vi "Handle Command.vi"(8 "error in (no error)":errorcluster, 9 "Data":variant, 10 "Command":string, 11 "Inst.Attocube-3DR in":refnum<class "Inst.Attocube-3DR.lvclass">) -> (0 "error out":errorcluster, 1 "Processed Data":variant, 2 "Command":string, 3 "Inst.Attocube-3DR out":refnum<class "Inst.Attocube-3DR.lvclass">)   [LabVIEW 2019, in "Inst.Attocube-3DR.lvclass"]
uses:
  Inst.Attocube-3DR.lvclass
  Inst.Attocube-3DR.lvclass/Inst.Attocube-3DR.ctl
  Typedefs/Inst.Attocube-3DR.getAll--Cluster.ctl
  9aec49fd-fe04-463a-be35-b7075f22e824.vi
  9aec49fd-fe04-463a-be35-b7075f22e824.vi/2713e523-c1ef-4f5d-940a-2c453df62ff4.vi
  9aec49fd-fe04-463a-be35-b7075f22e824.vi/a90875ce-4e03-4b08-b88d-0b37294445d5.vi
  <vilib>/Utility/Data Type/Get Type Information.vi
  <vilib>/JDP Science/JSONtext/JSON text to Variant.vi
  <vilib>/JDP Science/JSONtext/LVClass Serializer/JSONtext LVClass Serializer.lvclass
  <userlib>/LevyLab/Instrument Framework/Instrument Types/VSource/Instrument.VSource.lvclass
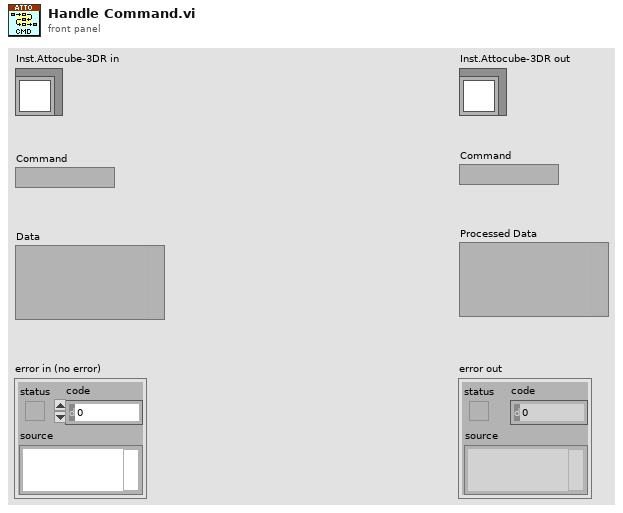
[diagram p1: front panel]
types:
  T1 = typedef "Inst.Attocube-3DR.lvclass/Inst.Attocube-3DR.getAll--Cluster.ctl" = cluster{"Axis 1: Amplitude":i32, "Axis 1: Capacitance":i32, "Axis 1: Current Position":i32, "Axis 1: DCLevel":i32, "Axis 1: Frequency":i32, "Axis 1: StepWidth":i32, "Axis 1: control mode":i32, "Axis 1: rot. count":i32, "Axis 1: sp position":i32, "Axis 1: sp rot. count":i32, "Axis 1: speed":i32, "Axis 1: Target GND":bool, "Axis 1: Output":bool, "Axis 1: Single Circle Mode":bool, "Axis 1: moving":bool, "Axis 1: stop detected":bool, "Axis 1:  sensor error":bool, "Axis 1: sensor diconnected":bool, "Axis 1: stop enable":bool, "Axis 2: Current Position":i32, "Axis 2: DCLevel":i32, "Axis 2: Frequency":i32, "Axis 2: StepWidth":i32, "Axis 2: control mode":i32, "Axis 2: rot. count":i32, "Axis 2: sp position":i32, "Axis 2: sp rot. count":i32, "Axis 2: speed":i32, "Axis 2: Capacitance":i32, "Axis 2: Amplitude":i32, "Axis 2: Target GND":bool, "Axis 2: Output":bool, "Axis 2: Single Circle Mode":bool, "Axis 2: moving":bool, "Axis 2: stop detected":bool, "Axis 2:  sensor error":bool, "Axis 2: sensor diconnected":bool, "Axis 2: stop enable":bool}
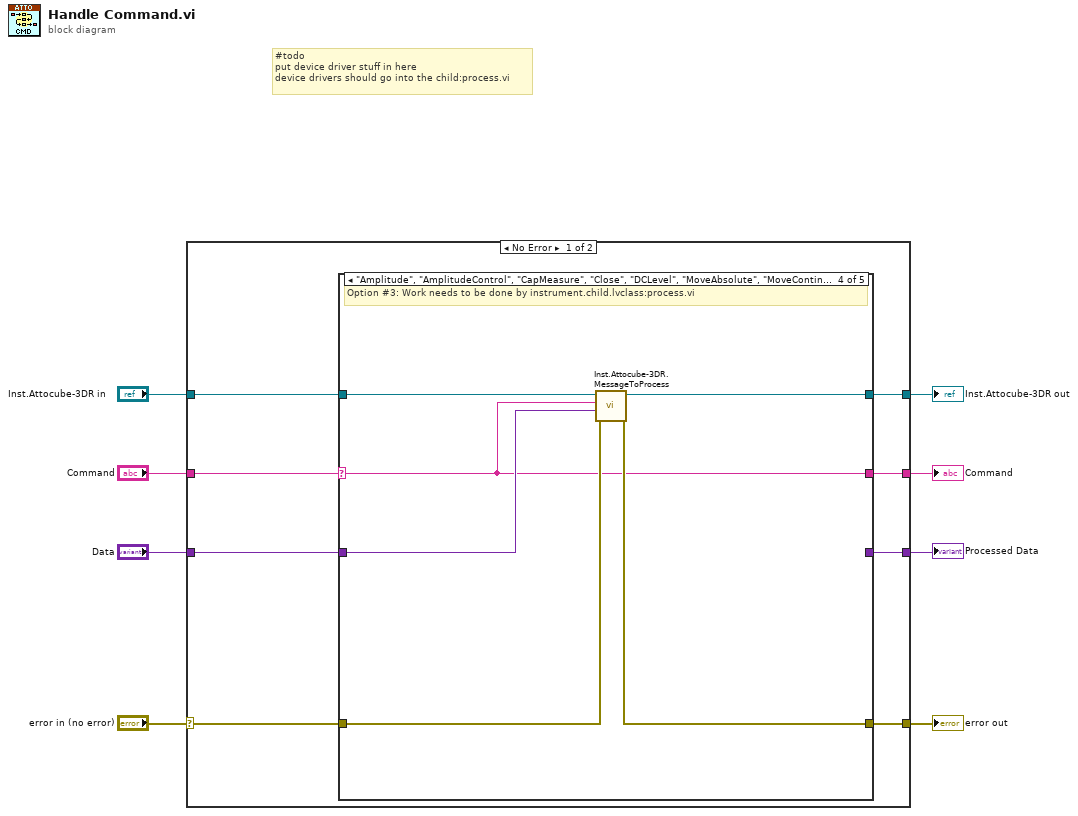
[diagram p0: block diagram]
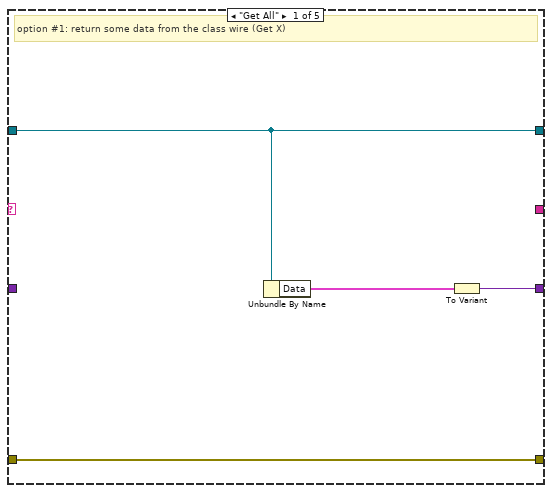
[diagram p2: hidden frame]
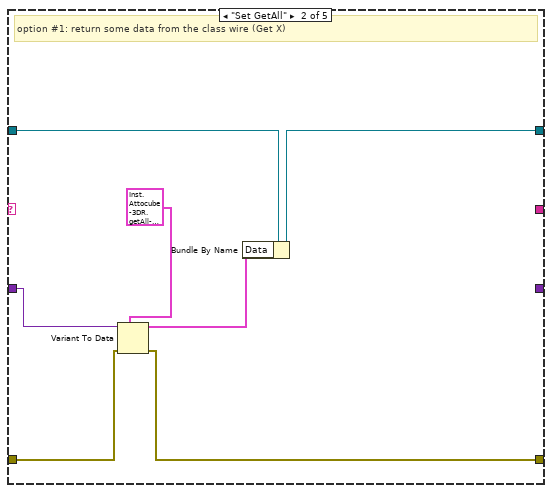
[diagram p3: hidden frame]
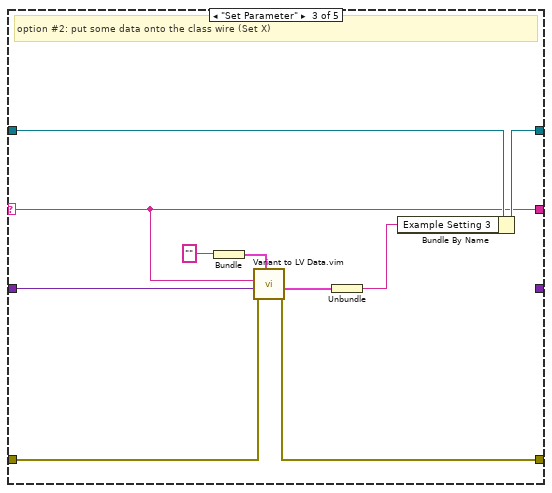
[diagram p4: hidden frame]
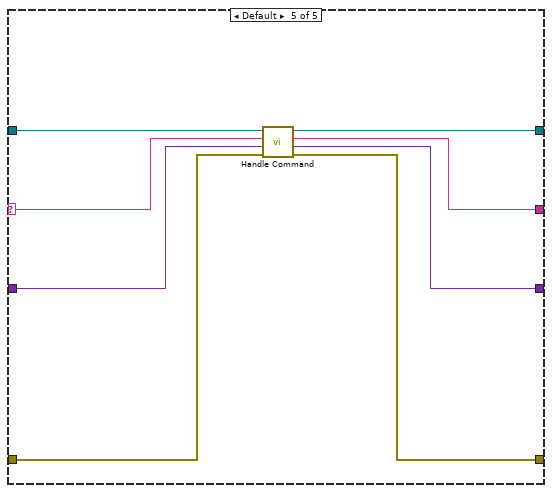
[diagram p5: hidden frame]
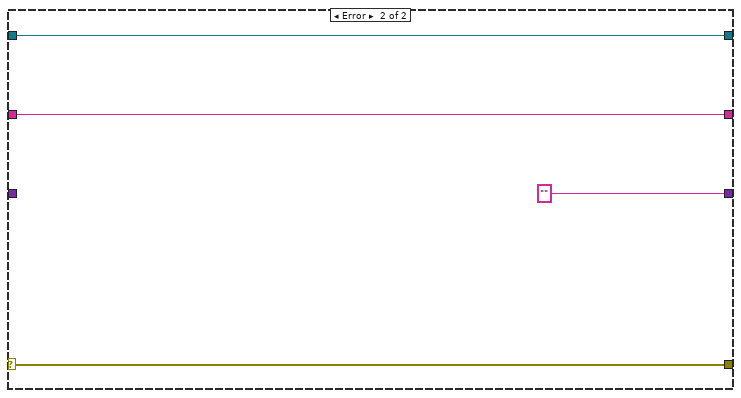
[diagram p6: hidden frame]
diagram:
  # "#todo\nput device driver stuff in here\ndevice drivers should go into the child:process.vi"
  n1 = case shown="No Error" "error in (no error)" {
    selector: "error in (no error)" -> [w10 w55]
    tunnel: [w12 w55] -> w6
    tunnel: [w14 w54] -> w5
    tunnel: "Inst.Attocube-3DR in" -> [w15 w54]
    tunnel: "Command" -> [w16 w52]
    tunnel: [w13 "" ("String")] -> w3
    tunnel: "Data" -> [w9 _]
    tunnel: [w11 w52] -> w1
    frame No Error {
      n2 = case shown="\"Amplitude\", \"AmplitudeControl\", \"CapMeasure\", \"Close\", \"DCLevel\", \"MoveAbsolute\", \"MoveContinuous\", \"MoveRelative\", \"MoveSingleStep\", \"Open\", \"SetOutput\", \"SetTargetGround\", \"SingleCircleMode\", \"StopDetection\", \"StopMoving\", \"setFrequency\"" w16 {
        selector: w16 -> [_ _ w32 w38 w45]
        tunnel: w15 -> [w19 w21 w37 w43 w49]
        tunnel: [w19 w22 w36 w42 w46] -> w14
        tunnel: [w17 _ _ _ w48] -> w13
        tunnel: w10 -> [w18 w26 w35 w41 w50]
        tunnel: w9 -> [_ w25 w33 w39 w51]
        tunnel: [w18 w27 w34 w40 w47] -> w12
        tunnel: [_ _ w32 w38 w44] -> w11
        frame "Get All" {
          # "option #1: return some data from the class wire (Get X)"
          n3 = Unbundle By Name(w19) -> ("Data"=w20:T1)
          n4 = To Variant(anything=w20) -> (Variant=w17:variant)
        }
        frame "Set GetAll" {
          # "option #1: return some data from the class wire (Get X)"
          n5 = Variant To Data(error in=w26, type=T1 {"Axis 1: Amplitude"=0, "Axis 1: Capacitance"=0, "Axis 1: Current Position"=0, "Axis 1: DCLevel"=0, "Axis 1: Frequency"=0, "Axis 1: StepWidth"=0, "Axis 1: control mode"=0, "Axis 1: rot. count"=0, "Axis 1: sp position"=0, "Axis 1: sp rot. count"=0, "Axis 1: speed"=0, "Axis 1: Target GND"=FALSE, "Axis 1: Output"=FALSE, "Axis 1: Single Circle Mode"=FALSE, "Axis 1: moving"=FALSE, "Axis 1: stop detected"=FALSE, "Axis 1:  sensor error"=FALSE, "Axis 1: sensor diconnected"=FALSE, "Axis 1: stop enable"=FALSE, "Axis 2: Current Position"=0, "Axis 2: DCLevel"=0, "Axis 2: Frequency"=0, "Axis 2: StepWidth"=0, "Axis 2: control mode"=0, "Axis 2: rot. count"=0, "Axis 2: sp position"=0, "Axis 2: sp rot. count"=0, "Axis 2: speed"=0, "Axis 2: Capacitance"=0, "Axis 2: Amplitude"=0, "Axis 2: Target GND"=FALSE, "Axis 2: Output"=FALSE, "Axis 2: Single Circle Mode"=FALSE, "Axis 2: moving"=FALSE, "Axis 2: stop detected"=FALSE, "Axis 2:  sensor error"=FALSE, "Axis 2: sensor diconnected"=FALSE, "Axis 2: stop enable"=FALSE} ("getAll"), Variant=w25) -> (data=w23:T1, error out=w27:errorcluster)
          n6 = Bundle By Name(cluster=w21, "Data"=w23) -> (w22:refnum<class "Inst.Attocube-3DR.lvclass">)
        }
        frame "Set Parameter" {
          # "option #2: put some data onto the class wire (Set X)"
          n7 = Bundle("") -> (w30:cluster{string})  [unwired: 1 in]
          n8 = call "Variant to LV Data.vim"("type"=w30, "error in (no error)"=w35, "JSON Data in"=w33, "Command"=w32) -> ("error out"=w34:errorcluster, "Data out"=w29:cluster{string})  [unwired: 4 in, 2 out]
          n9 = Unbundle(w29) -> (w28:string)
          n10 = Bundle By Name(cluster=w37, "Example Setting 3"=w28) -> (w36:refnum<class "Inst.Attocube-3DR.lvclass">)
        }
        frame "Amplitude", "AmplitudeControl", "CapMeasure", "Close", "DCLevel", "MoveAbsolute", "MoveContinuous", "MoveRelative", "MoveSingleStep", "Open", "SetOutput", "SetTargetGround", "SingleCircleMode", "StopDetection", "StopMoving", "setFrequency" {
          # "Option #3: Work needs to be done by instrument.child.lvclass:process.vi"
          n11 = call "Inst.Attocube-3DR.MessageToProcess.vi"("error in (no error)"=w41, "Data"=w39, "Command"=w38, "Inst.Attocube-3DR in"=w43) -> ("error out"=w40:errorcluster, "Inst.Attocube-3DR out"=w42:refnum<class "Inst.Attocube-3DR.lvclass">)  [unwired: 6 in]
        }
        frame Default {
          n12 = call-parent "Handle Command.vi"("error in (no error)"=w50, "Data"=w51, "Command"=w45, "Instrument in"=w49) -> ("error out"=w47:errorcluster, "Processed Data"=w48:variant, "Command"=w44:string, "Instrument out"=w46:refnum<class "Inst.Attocube-3DR.lvclass">)  [unwired: 4 in]
        }
      }
    }
    frame Error {
    }
  }
  "error out" <- w6
  "Inst.Attocube-3DR out" <- w5
  "Command" <- w1
  "Processed Data" <- w3
